vi "CONTROL ARM STROKE.vi"(0 "refnum name":string="ClimberRIGHT", 1 "PID gains":T1={"proportional gain (Kc)"=0.05, "integral time (Ti, min)"=0.05, "derivative time (Td, min)"=0.006} {"derivative time (Td, min)" format="%.3f"; "integral time (Ti, min)" format="%.3f"; "proportional gain (Kc)" format="%.6f"}, 2 "output range":cluster{"output high":dbl, "output low":dbl}={"output high"=0.75, "output low"=-0.75} {"output low" format="%.2f"; "output high" format="%.2f"}, 5 "setpoint (in)":dbl(slide)=20.0 min=0.0 max=22.0 scale=0.0..22.0, 7 "error tolerance (in)":dbl=0.25 format="%#_13g", 9 "times within tolerance":i32=6, 12 "reinitialize? (F)":bool=TRUE, 13 "invert sensor?":bool) -> (8 "position (in)":dbl=20.046974932675433, 10 "setpoint error (in)":dbl=-0.04697493267543481)   [LabVIEW 2020]
uses:
  <vilib>/Rock Robotics/WPI/ThirdParty/Phoenix-LabVIEW/Motor Controller/Controls/CTRE_Phoenix_MotorControl_ControlMode.ctl
  Robot Global Data.vi
  <vilib>/Rock Robotics/Network Tables/NT Write Boolean.vi
  <vilib>/Rock Robotics/WPI/ThirdParty/Phoenix-LabVIEW/Motor Controller/Get/CTRE_Phoenix_MotorController_IntegratedSensorData_TalonFX.vi
  <vilib>/addons/control/pid/pid.llb/PID (DBL).vi
  <vilib>/Rock Robotics/WPI/ThirdParty/Phoenix-LabVIEW/Motor Controller/Get/CTRE_Phoenix_MotorController_GetSelectedSensorData.vi
  <vilib>/addons/control/pid/NI_PID_pid.lvlib
panel:
  out "x > y?":bool=TRUE
  out "output":dbl=-0.75 format="%.2f"
  out "Position":dbl=364705.0 format="%.2f"
  out "Position (Raw Sensor Units)":i32=351863
  out "setpoint 2":dbl=20.0
  out "Chart set point & postition 2":cluster{"setpoint":dbl, dbl}(graph)={"setpoint"=363850.40758, 364705.0}
  in  "stop":bool
  out "setpoint error (tics)":dbl=-854.5924200000009
  out "Chart motor output":dbl(graph)=-0.75
  out "Chart set point & postition":cluster{"setpoint":dbl, dbl}(graph)={"setpoint"=20.0, 20.046974932675433}
  # "scale 40% @ 2in\n100% @ >5\" error"
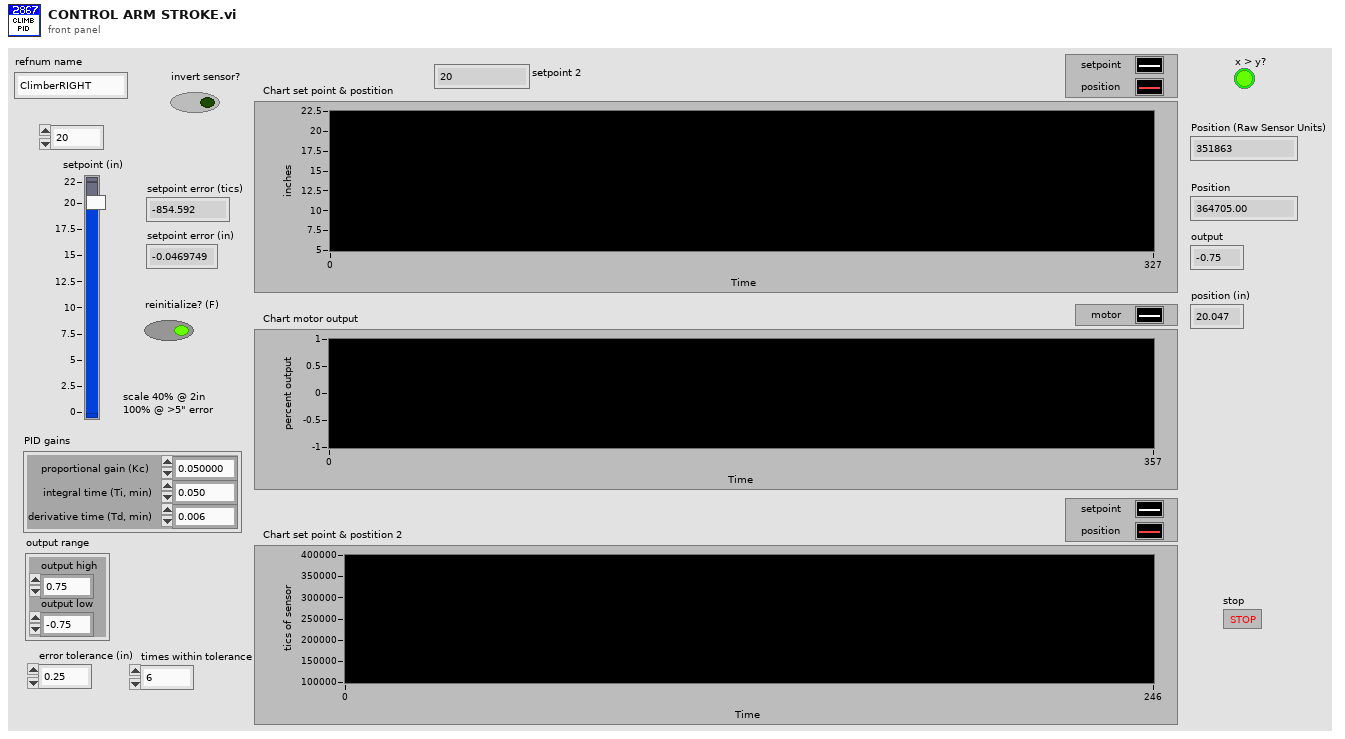
[diagram p1: front panel]
types:
  T1 = cluster{"proportional gain (Kc)":dbl, "integral time (Ti, min)":dbl, "derivative time (Td, min)":dbl}
  T2 = typedef "CTRE_Phoenix_MotorControl_ControlMode.ctl" = u16
  T3 = typedef "WPI_MotorControlDeviceRef.ctl" = cluster{"DeviceStatus":errorcluster, "Type":T4, "PWM":cluster{"PWM Channel":T5, "DeadBand":T6}, "CAN":cluster{"Device Number":u8, "SetOutput VI Ref":variant, "GetOutput VI Ref":variant, "Enable VI Ref":variant, "Disable VI Ref":variant, "Data":variant}, "Invert":bool, "DIO PWM":cluster{"PWM \"Enable\" Channel":T5, "DIOChannel":T7, "PWM Rate":dbl}}
  T4 = typedef "WPI_MotorControlType.ctl" = enum16{"PWM", "CAN", "DIO PWM"}
  T5 = typedef "FPGA_DIOPWMChannel.ctl" = enum8{"PWM 0", "PWM 1", "PWM 2", "PWM 3", "PWM 4", "PWM 5", "PWM 6", "PWM 7", "PWM 8", "PWM 9", "PWM MXP 0", "PWM MXP 1", "PWM MXP 2", "PWM MXP 3", "PWM MXP 4", "PWM MXP 5", "PWM MXP 6", "PWM MXP 7", "PWM MXP 8", "PWM MXP 9", "Invalid"}
  T6 = typedef "WPI_PWMDeadband.ctl" = cluster{"Name":string, "maxPositivePwm":i32, "minPositivePwm":i32, "centerPwm":i32, "maxNegativePwm":i32, "minNegativePwm":i32, "angularRange":u16}
  T7 = typedef "FPGA_DIOChannel.ctl" = enum8{"DIO 0", "DIO 1", "DIO 2", "DIO 3", "DIO 4", "DIO 5", "DIO 6", "DIO 7", "DIO 8", "DIO 9", "DIO MXP 0", "DIO MXP 1", "DIO MXP 2", "DIO MXP 3", "DIO MXP 4", "DIO MXP 5", "DIO MXP 6", "DIO MXP 7", "DIO MXP 8", "DIO MXP 9", "DIO MXP 10", "DIO MXP 11", "DIO MXP 12", "DIO MXP 13", "DIO MXP 14", "DIO MXP 15", "SPI Port CS1", "SPI Port CS2", "SPI Port CS3", "SPI Port MISO", "SPI Port MOSI", "Invalid"}
  T8 = cluster{"MIN":dbl, "MAX":dbl, "convert climber inches to tics":dbl, "INITIALIZE":dbl}
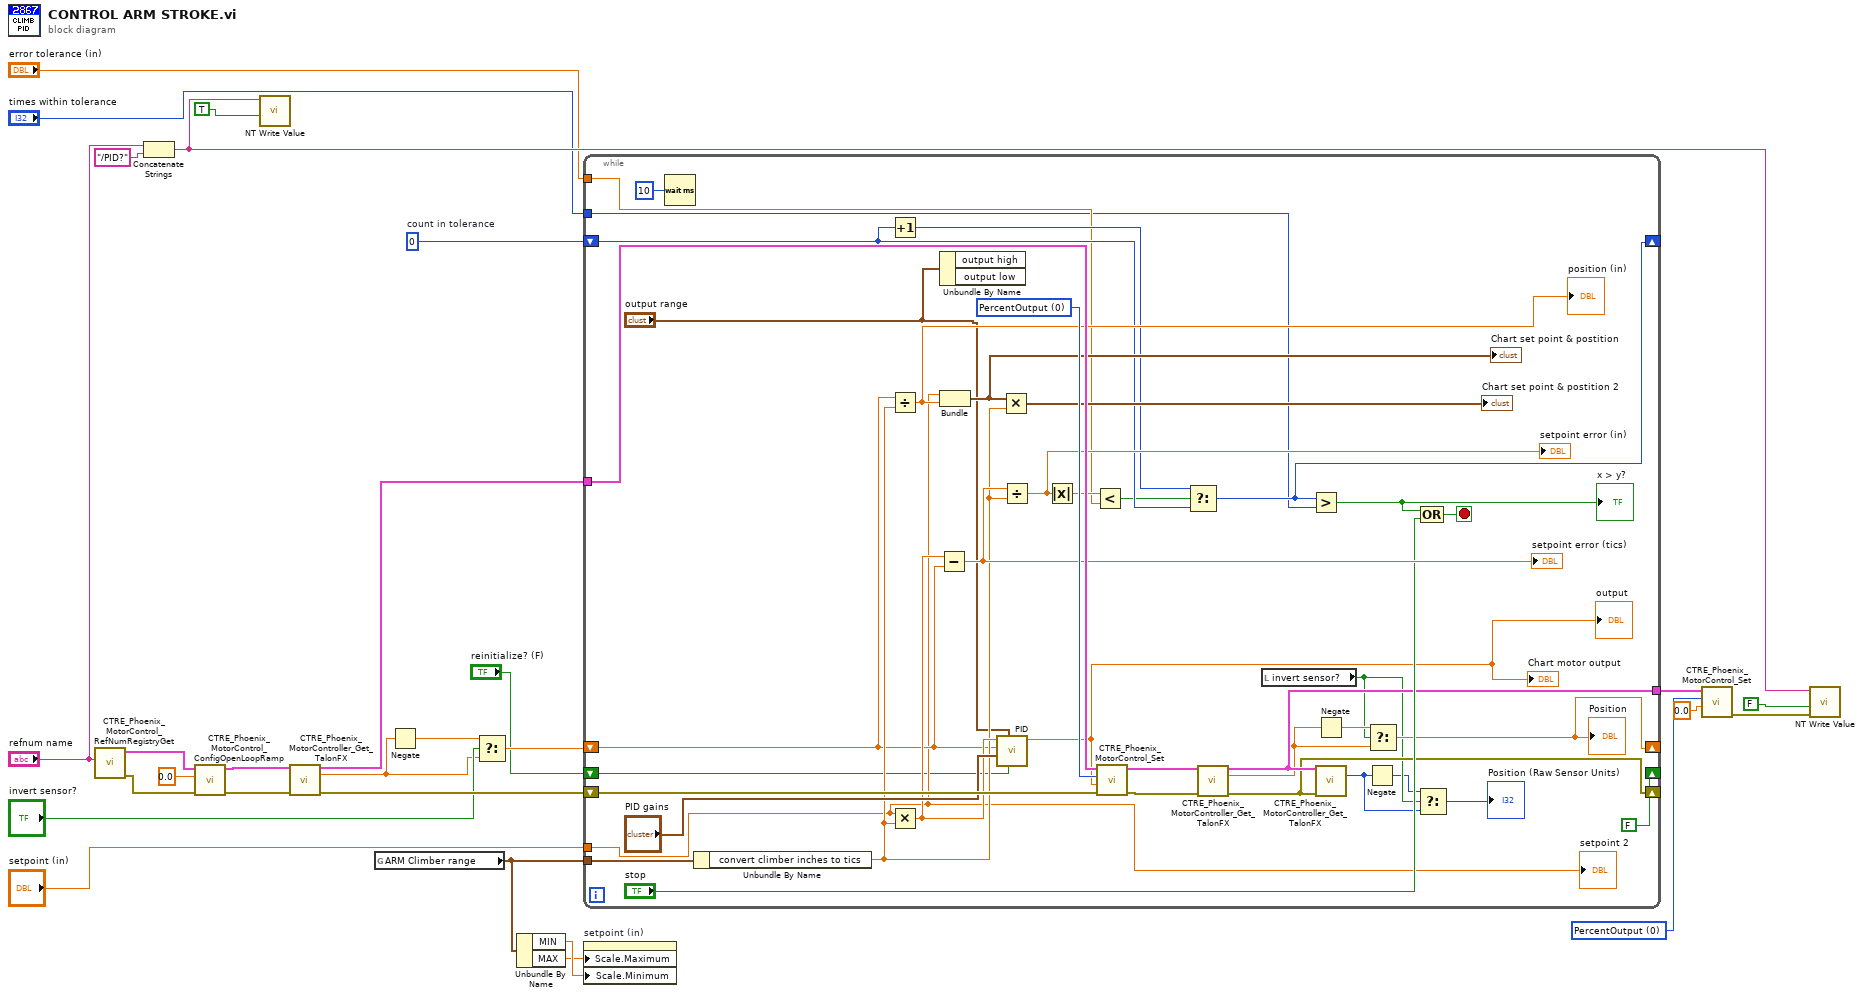
[diagram p0: block diagram]
diagram:
  w8 = 0  # count in tolerance
  w13 = T2 0 items=["PercentOutput"=0, "Position"=1, "Velocity"=2, "Current"=3, "Follower"=5, "MotionProfile"=6, "MotionMagic"=7, "MotionProfileArc"=10, "Disabled"=15] ("Control Mode")
  n1 = call <vilib>:"CTRE_Phoenix_MotorControl_RefNumRegistryGet.vi"("refnum name"="refnum name") -> ("error out"=w23:errorcluster, "PhoenixMotorControlDevRef"=w28:T3)  [unwired: 9 in]
  n2 = Concatenate Strings("refnum name", "/PID?" ("string")) -> (w15:string)
  n3 = call <vilib>:"CTRE_Phoenix_MotorControl_ConfigOpenLoopRamp.vi"("error in (no error)"=w23, "secondsFromNeutralToFull"=0.0, "PhoenixMotorControlDevRef"=w28) -> ("error out"=w22:errorcluster, "PhoenixMotorControlDevRef"=w25:T3)  [unwired: 7 in]
  n4 = call-poly <vilib>:"NT Write Value.vi"("Boolean"=TRUE, "Name"=w15) -> ()  [unwired: 9 in, 1 out]
  n5 = call-poly <vilib>:"CTRE_Phoenix_MotorController_Get_TalonFX.vi"("PhoenixMotorControlDevRef"=w25, "error in"=w22) -> ("PhoenixMotorControlDevRef"=w27:T3, "Position"=w3:dbl, "error out"=w26:errorcluster)  [unwired: 9 in, 2 out]
  n6 = global read "Robot Global Data.vi" "ARM Climber range"() -> (w21:T8)
  n7 = Negate(x=w3) -> (-x=w2:dbl)
  n8 = Select(t=w2, s="invert sensor?", f=w3) -> (s? t:f=w5:dbl)
  n9 = Unbundle By Name(w21) -> ("MIN"=w20:dbl, "MAX"=w19:dbl)
  n10 = while {
    tunnel: w21 -> [w67]
    tunnel: w27 -> [w68]
    shift-right: [w37] -> _
    shift-left: w5 -> [w53]
    shift-right: [w48] -> _
    shift-left: w26 -> [w64]
    tunnel: [w51] -> w14
    tunnel: "setpoint (in)" -> [w47]
    shift-right: [w41] -> _
    shift-left: w8 -> [w44]
    tunnel: "error tolerance (in)" -> [w39]
    tunnel: "times within tolerance" -> [w38]
    shift-right: [FALSE ("reinitialize? (F)")] -> _
    shift-left: "reinitialize? (F)" -> [w30]
    stop <- w54 stop-if-true
    w65 = T2 0 items=["PercentOutput"=0, "Position"=1, "Velocity"=2, "Current"=3, "Follower"=5, "MotionProfile"=6, "MotionMagic"=7, "MotionProfileArc"=10, "Disabled"=15] ("Control Mode")
    n11 = Wait (ms)(milliseconds to wait=u32 10) -> ()  [unwired: 1 out]
    n12 = Unbundle By Name(w67) -> ("convert climber inches to tics"=w56:dbl)
    n13 = Increment(x=w44) -> (x+1=w42:i32)
    n14 = Divide(x=w53, y=w56) -> (x/y=w59:dbl)
    "position (in)" <- w59
    n15 = Multiply(x=w47, y=w56) -> (x*y=w61:dbl)
    n16 = Subtract(x=w61, y=w53) -> (x-y=w60:dbl)
    "setpoint error (tics)" <- w60
    n17 = Unbundle By Name("output range") -> ()  [unwired: 2 out]
    n18 = Bundle("setpoint (in)"=w47, w59) -> (w58:cluster{"setpoint (in)":dbl, dbl})  [unwired: 1 in]
    "Chart set point & postition" <- w58
    n19 = call-poly <vilib>:"PID.vi"("reinitialize? (F)"=w30, "output range"="output range", "PID gains"="PID gains", "process variable"=w53, "setpoint"=w61) -> ("output"=w49:dbl)  [unwired: 5 in, 1 out]
    "Chart motor output" <- w49
    "output" <- w49
    n20 = Multiply(x=w58, y=w56) -> (x*y=→"Chart set point & postition 2":cluster{"setpoint (in)":dbl, dbl})
    n21 = Divide(x=w60, y=w56) -> (x/y=w46:dbl)
    "setpoint error (in)" <- w46
    n22 = Absolute Value(x=w46) -> (abs(x)=w45:dbl)
    n23 = Less?(x=w45, y=w39) -> (x < y?=w43:bool)
    n24 = call <vilib>:"CTRE_Phoenix_MotorControl_Set.vi"("error in (no error)"=w64, "Output"=w49, "Control Mode"=w65, "PhoenixMotorControlDevRef"=w68) -> ("error out"=w63:errorcluster, "PhoenixMotorControlDevRef"=w66:T3)  [unwired: 6 in]
    n25 = Select(t=w42, s=w43, f=w44) -> (s? t:f=w41:i32)
    n26 = call-poly <vilib>:"CTRE_Phoenix_MotorController_Get_TalonFX.vi"("PhoenixMotorControlDevRef"=w66, "error in"=w63) -> ("PhoenixMotorControlDevRef"=w51:T3, "Position"=w36:dbl, "error out"=w48:errorcluster)  [unwired: 9 in, 2 out]
    n27 = local read "invert sensor?"() -> (w32:bool)
    n28 = Greater?(x=w41, y=w38) -> (0:w40:bool)
    "x > y?" <- w40
    n29 = Negate(x=w36) -> (-x=w35:dbl)
    n30 = call-poly <vilib>:"CTRE_Phoenix_MotorController_Get_TalonFX.vi"("PhoenixMotorControlDevRef"=w51, "error in"=w48) -> ("Position (Raw Sensor Units)"=w33:i32)  [unwired: 10 in, 3 out]
    n31 = Negate(x=w33) -> (-x=w31:i32)
    n32 = Select(t=w35, s=w32, f=w36) -> (s? t:f=w37:dbl)
    "Position" <- w37
    n33 = Select(t=w31, s=w32, f=w33) -> (s? t:f=→"Position (Raw Sensor Units)":i32)
    n34 = Compound Arithmetic op=OR(w40, "stop") -> (w54:bool)
    "setpoint 2" <- w47
  }
  n35 = property on="setpoint (in)" class="Slide (strict)"("Scale.Maximum"=w19, "Scale.Minimum"=w20) -> ()  [unwired: 2 in, 2 out]
  n36 = call <vilib>:"CTRE_Phoenix_MotorControl_Set.vi"("Output"=0.0, "Control Mode"=w13, "PhoenixMotorControlDevRef"=w14) -> ("error out"=w10:errorcluster)  [unwired: 7 in, 1 out]
  n37 = call-poly <vilib>:"NT Write Value.vi"("error in"=w10, "Boolean"=FALSE, "Name"=w15) -> ()  [unwired: 8 in, 1 out]
